vi "Read Rigid Body Data.vi"(8 "error in (no error)":errorcluster, 11 "Tracking Data In":T1) -> (0 "error out":errorcluster, 3 "Tracking Data Out":T1)   [LabVIEW 2017]
uses:
  Controls/Rigid Body Info.ctl
  Controls/Position.ctl
  Controls/Orientation.ctl
  Controls/Tracking Data.ctl
  Controls/Packet Data.ctl
  Controls/Tracker Type.ctl
panel:
  out "return count":u32
  out "read buffer":string
  out "Rigid Body Data":T3
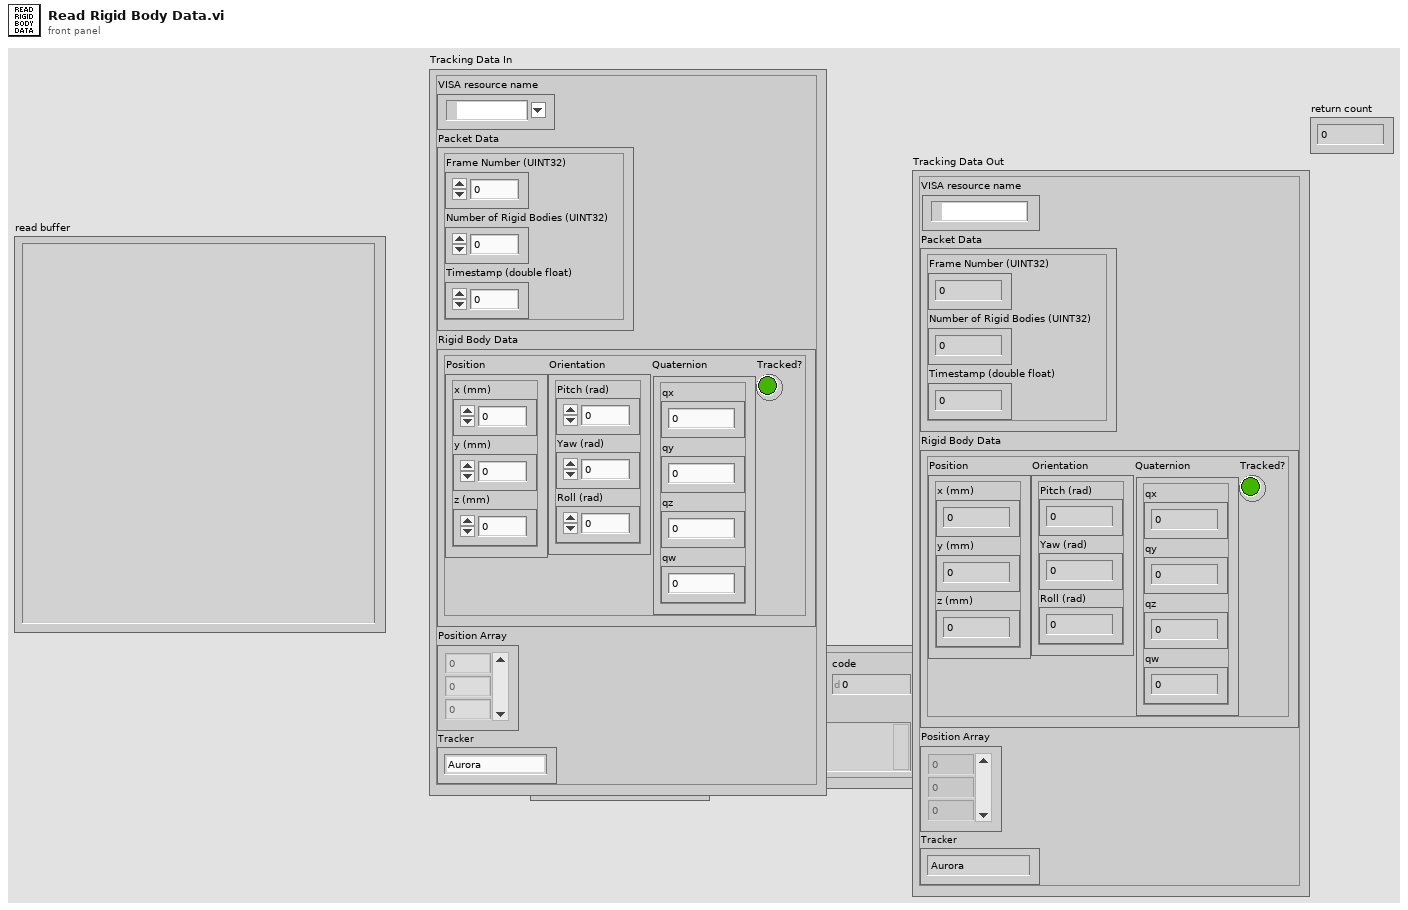
[diagram p1: front panel]
types:
  T1 = typedef "Tracking Data.ctl" = cluster{"VISA resource name":refnum<visa-resource-name>, "Packet Data":T2, "Rigid Body Data":T3, "Position Array":dbl[][], "Tracker":T6}
  T2 = typedef "Packet Data.ctl" = cluster{"Frame Number (UINT32)":u32, "Number of Rigid Bodies (UINT32)":u32, "Timestamp (double float)":dbl}
  T3 = typedef "Rigid Body Info.ctl" = cluster{"Position":T4, "Orientation":T5, "Quaternion":cluster{"qx":sgl, "qy":sgl, "qz":sgl, "qw":sgl}, "Tracked?":bool}
  T4 = typedef "Position.ctl" = cluster{"x (mm)":sgl, "y (mm)":sgl, "z (mm)":sgl}
  T5 = typedef "Orientation.ctl" = cluster{"Pitch (rad)":sgl, "Yaw (rad)":sgl, "Roll (rad)":sgl}
  T6 = typedef "Tracker Type.ctl" = enum16{"Aurora", "OptiTrack"}
  T7 = typedef "Raw Rigid Body Data.ctl" = cluster{"Body ID (UINT32)":u32, "x (single float)":sgl, "y (single float)":sgl, "z (single float)":sgl, "qx (single float)":sgl, "qy (single float)":sgl, "qz (single float)":sgl, "qw (single float)":sgl, "Tracked 1 (UINT8)":u8, "Tracked 2 (UINT8)":u8}
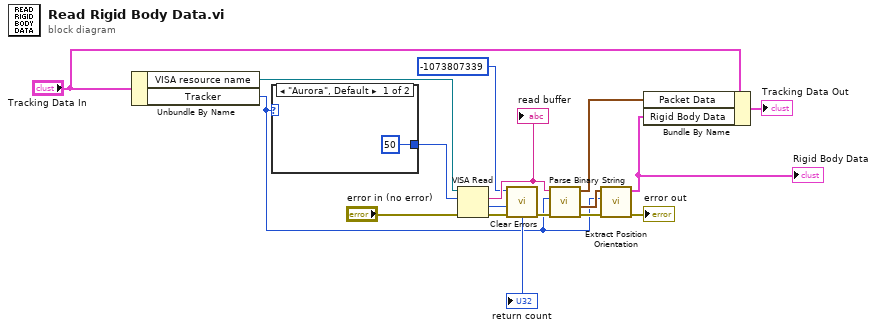
[diagram p0: block diagram]
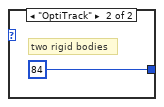
[diagram p2: hidden frame]
diagram:
  n1 = Unbundle By Name("Tracking Data In") -> ("VISA resource name"=w7:refnum<visa-resource-name>, "Tracker"=w1:T6)
  n2 = case shown="\"Aurora\", Default" w1 {
    tunnel: [u32 50 ("byte count") u32 84 ("byte count")] -> w11
    frame "Aurora", Default {
    }
    frame "OptiTrack" {
      # "two rigid bodies"
    }
  }
  n3 = VISA Read(VISA resource name=w7, byte count=w11, error in (no error)="error in (no error)") -> (read buffer=w12:string, return count=→"return count":u32, error out=w10:errorcluster)  [unwired: 1 out]
  "read buffer" <- w12
  n4 = call <vilib>:"Clear Errors.vi"("error in (no error)"=w10, "specific error code to clear (0: all)"=-1073807339) -> ("error out"=w13:errorcluster)  [unwired: 4 in, 1 out]
  n5 = call "Parse Binary String.vi"("Error In"=w13, "Tracker"=w1, "read buffer in"=w12) -> ("Error Out"=w15:errorcluster, "Rigid Body Data"=w14:T7[], "Packet Data"=w5:T2)  [unwired: 5 in, 1 out]
  n6 = call "Extract Position Orientation.vi"("Error In"=w15, "Tracker"=w1, "Rigid Body Data"=w14) -> ("Error Out"=→"error out":errorcluster, "Rigid Body"=w4:T3)  [unwired: 7 in]
  "Rigid Body Data" <- w4
  n7 = Bundle By Name(cluster="Tracking Data In", "Packet Data"=w5, "Rigid Body Data"=w4) -> (→"Tracking Data Out":T1)
